vi "SetVoltage.vi"(2 "Voltage":dbl, 3 "Name":string) -> (0 "Reply":string, 1 "Error":bool)   [LabVIEW 2014]
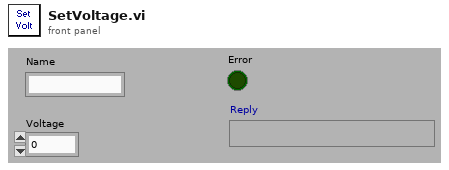
[diagram p1: front panel]
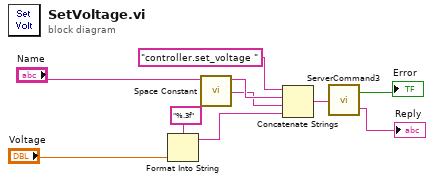
[diagram p0: block diagram]
diagram:
  n1 = Format Into String(format string="%.3f", "Voltage") -> (resulting string=w6:string)  [unwired: 2 in, 1 out]
  n2 = call <vilib>:"Space Constant.vi"() -> ("String"=w1:string)
  n3 = Concatenate Strings("controller.set_voltage " ("Command"), "Name", w1, w6) -> (w9:string)
  n4 = call "ServerCommand3.vi"("Command"=w9) -> ("Error"=→"Error":bool, "Reply"=→"Reply":string)
